vi "tool_Unicode_Convert Unicode to ANSI.vi"(7 "Dest. Code Page":T1 items=["System Default"=0, "Thai"=874, "Japanese"=932, "Chinese - Simplified"=936, "Korean"=949, "Chinese - Traditional"=950, "Central Europe"=1250, "Cyrillic"=1251, "Western Europe - Latin"=1252, "Greek"=1253, "Turkish"=1254, "Hebrew"=1255, "Arabic"=1256, "Baltic"=1257, "Vietnamese"=1258, "Unicode UTF-8"=65001], 10 "error in (no error)":errorcluster, 11 "WideChar (UTF16-LE)":string) -> (2 "error out":errorcluster, 3 "MultiByteStr (ANSI)":string)   [LabVIEW 2013, in "SET_Unicode Tools.lvlib"]
doc: "tool_Unicode_Convert Unicode to ANSI.vi\n\nConvert UTF-16LE string to Multi-Byte String of a specified code page.\nDefault code page is the system's active code page.\n \nThis function calls WideCharToMultiByte from kernel32.dll"
uses:
  SET_Unicode Tools.lvlib
  Code Page List.ctl
  kernel32.dll
panel:
  out "NumBytes":i32
  # "tool_Unicode_Convert Unicode to ANSI.vi\n\nConvert UTF-16LE string to Multi-Byte String of a specified code page.\nDefault code page is the system's active code page.\n \nThis function calls WideCharToMultiByte from kernel32.dll"
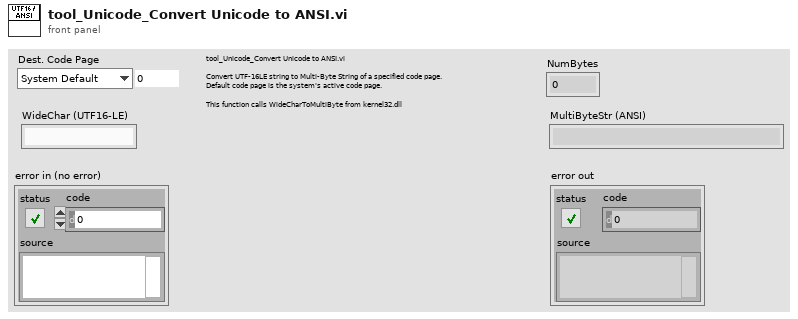
[diagram p1: front panel]
types:
  T1 = typedef "SET_Unicode Tools.lvlib/Code Page List.ctl" = u16
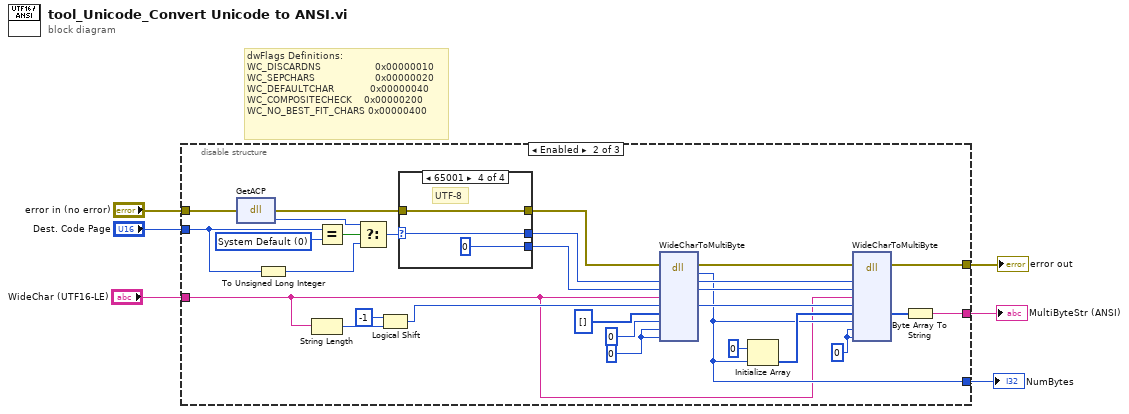
[diagram p0: block diagram]
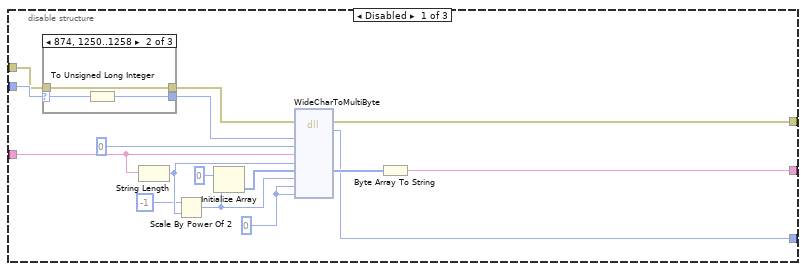
[diagram p2: hidden frame]
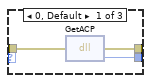
[diagram p3: hidden frame]
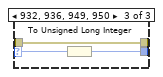
[diagram p4: hidden frame]
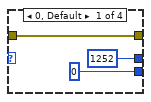
[diagram p5: hidden frame]
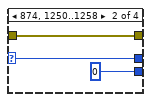
[diagram p6: hidden frame]
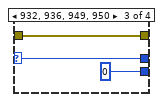
[diagram p7: hidden frame]
diagram:
  # "dwFlags Definitions:\nWC_DISCARDNS                  0x00000010\nWC_SEPCHARS                    0x00000020\nWC_DEFAULTCHAR            0x00000040\nWC_COMPOSITECHECK    0x00000200\nWC_NO_BEST_FIT_CHARS 0x00000400"
  n1 = disable-structure shown="Enabled" {
    disable-tunnel: "WideChar (UTF16-LE)" -> [w14 w32 _]
    disable-tunnel: "Dest. Code Page" -> [w13 w50 _]
    disable-tunnel: "error in (no error)" -> [w10 w51 _]
    disable-tunnel: [w9 w41 _] -> w3
    disable-tunnel: [w8 w58 _] -> w2
    disable-tunnel: [w7 w33 _] -> w1
    frame Disabled {
      w15 = u32 0
      n2 = case shown="874, 1250..1258" w13 {
        selector: w13 -> [_ w28 w31]
        tunnel: [w25 w27 w30] -> w12
        tunnel: w10 -> [w24 w26 w29]
        tunnel: [w23 w26 w29] -> w11
        frame 0, Default {
          n3 = dll-call lib="kernel32.dll" fn="GetACP" label="GetACP()"(error in=w24) -> (error out=w23:errorcluster, w25:u32)  [unwired: 2 in, 1 out]
        }
        frame 874, 1250..1258 {
          n4 = To Unsigned Long Integer(number=w28) -> (unsigned 32bit integer=w27:u32)
        }
        frame 932, 936, 949, 950 {
          n5 = To Unsigned Long Integer(number=w31) -> (unsigned 32bit integer=w30:u32)
        }
      }
      n6 = String Length(string=w14) -> (length=w18:i32)
      n7 = Scale By Power Of 2(n=-1, x=w18) -> (x*2^n=w16:i32)
      n8 = Initialize Array(u8 0, w16) -> (w21:u8[])
      n9 = dll-call lib="kernel32.dll" fn="WideCharToMultiByte"(error in=w11, "codePage"=w12, "dwFlags"=u32 0, "lpWideCharStr"=w14, "cchWideChar"=w18, "lpMultiByteStr"=w21, "cbMultiByte"=w16, "lpDefaultChar"=w15, "lpUsedDefaultChar"=w15) -> (error out=w9:errorcluster, "return type"=w7:i32, "lpMultiByteStr"=w22:u8[])  [unwired: 9 in, 1 out]
      n10 = Byte Array To String(unsigned byte array=w22) -> (string=w8:string)
    }
    frame Enabled {
      w34 = u32 0 ("lpUsedDefaultChar")
      w52 = T1 0 items=["System Default"=0, "Thai"=874, "Japanese"=932, "Chinese - Simplified"=936, "Korean"=949, "Chinese - Traditional"=950, "Central Europe"=1250, "Cyrillic"=1251, "Western Europe - Latin"=1252, "Greek"=1253, "Turkish"=1254, "Hebrew"=1255, "Arabic"=1256, "Baltic"=1257, "Vietnamese"=1258, "Unicode UTF-8"=65001] ("y")
      w59 = u32 0
      n11 = dll-call lib="kernel32.dll" fn="GetACP" label="GetACP()"(error in=w51) -> (error out=w57:errorcluster, w55:u32)  [unwired: 2 in, 1 out]
      n12 = To Unsigned Long Integer(number=w50) -> (unsigned 32bit integer=w56:u32)
      n13 = String Length(string=w32) -> (length=w46:i32)
      n14 = Equal?(x=w50, y=w52) -> (x = y?=w54:bool)
      n15 = Select(t=w55, s=w54, f=w56) -> (s? t:f=w53:u32)
      n16 = Logical Shift(y=-1 ("n"), x=w46) -> (x << y=w44:i32)
      n17 = case shown="65001" w53 {
        selector: w53 -> [_ w65 w68 w71]
        tunnel: [u32 1252 w65 w68 w71] -> w49
        tunnel: w57 -> [w63 w66 w69 w72]
        tunnel: [w63 w66 w69 w72] -> w48
        tunnel: [u32 0 ("MB_PRECOMPOSED") u32 0 ("MB_PRECOMPOSED") u32 0 ("MB_PRECOMPOSED") u32 0 ("NONE")] -> w47
        frame 0, Default {
        }
        frame 874, 1250..1258 {
        }
        frame 932, 936, 949, 950 {
        }
        frame 65001 {
          # "UTF-8"
        }
      }
      n18 = dll-call lib="kernel32.dll" fn="WideCharToMultiByte"(error in=w48, "codePage"=w49, "dwFlags"=w47, "lpWideCharStr"=w32, "cchWideChar"=w44, "lpMultiByteStr"=u8[] [], "cbMultiByte"=0, "lpDefaultChar"=w59, "lpUsedDefaultChar"=w59) -> (error out=w37:errorcluster, "return type"=w33:i32, "codePage"=w38:u32, "dwFlags"=w36:u32, "cchWideChar"=w35:i32)  [unwired: 7 in, 1 out]
      n19 = Initialize Array(u8 0, w33) -> (w39:u8[])
      n20 = dll-call lib="kernel32.dll" fn="WideCharToMultiByte"(error in=w37, "codePage"=w38, "dwFlags"=w36, "lpWideCharStr"=w32, "cchWideChar"=w35, "lpMultiByteStr"=w39, "cbMultiByte"=w33, "lpDefaultChar"=w34, "lpUsedDefaultChar"=w34) -> (error out=w41:errorcluster, "lpMultiByteStr"=w40:u8[])  [unwired: 9 in, 2 out]
      n21 = Byte Array To String(unsigned byte array=w40) -> (string=w58:string)
    }
    frame Disabled {
    }
  }
  "error out" <- w3
  "MultiByteStr (ANSI)" <- w2
  "NumBytes" <- w1
